vi "_list_CSM documented VIs.vi"(11 "Only CSM Folder":bool=TRUE) -> (3 "Array":path[](array[path]))   [LabVIEW 2017, in "csmdoc.lvlib"]
uses:
  csmdoc.lvlib
  _Shared/CSM Shared.lvlib
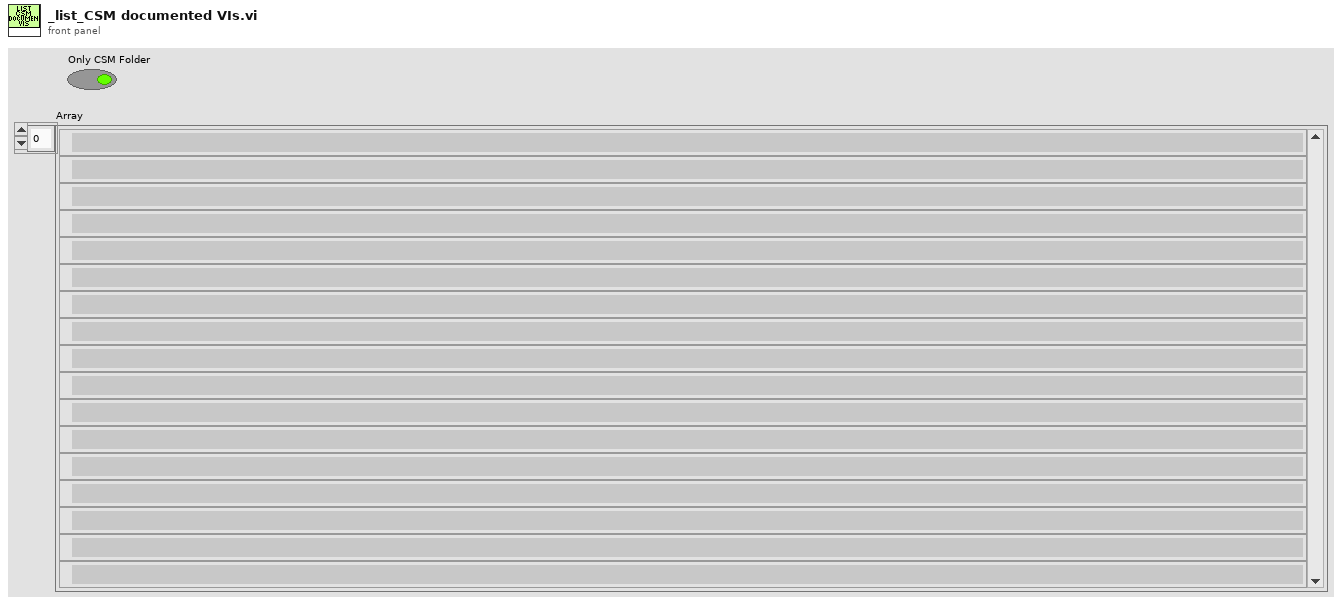
[diagram p1: front panel]
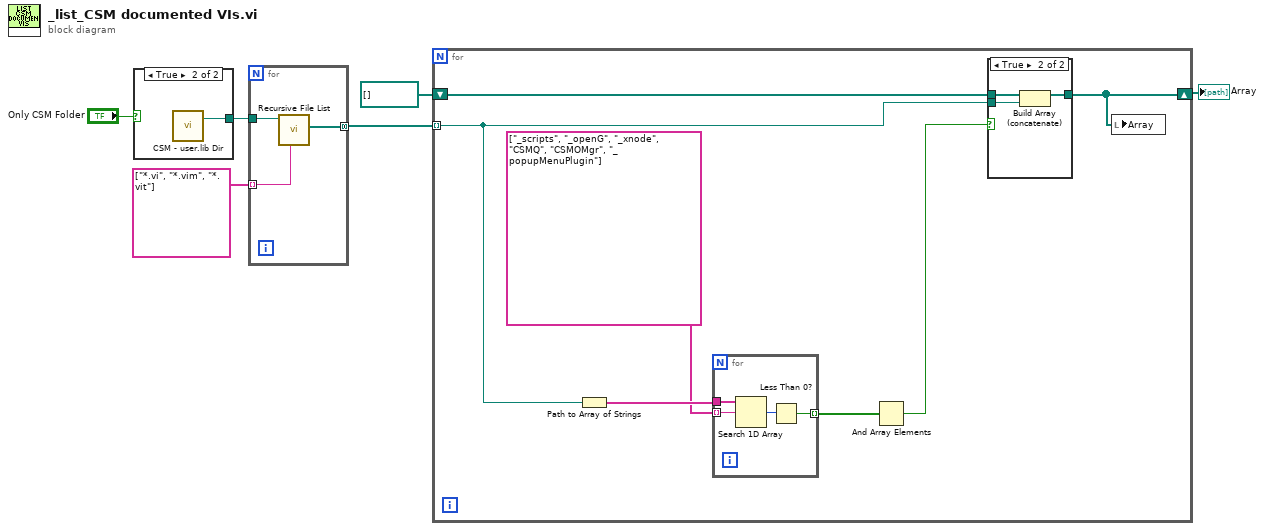
[diagram p0: block diagram]
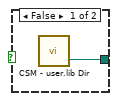
[diagram p2: hidden frame]
diagram:
  n1 = case shown="True" "Only CSM Folder" {
    tunnel: [w7 w8] -> w4
    frame False {
      n2 = call "CSM - user.lib Dir.vi"() -> ("<LabVIEW>"=w7:path)  [unwired: 2 in, 1 out]
    }
    frame True {
      n3 = call "CSM - user.lib Dir.vi"() -> ("csm_user.lib_dir"=w8:path)  [unwired: 2 in, 1 out]
    }
  }
  n4 = for {
    tunnel: w4 -> [w11]
    tunnel: string[] ["*.vi", "*.vim", "*.vit"] -> [w10] mode=indexing
    tunnel: [w9] -> w5 mode=concatenating
    n5 = call <vilib>:"Recursive File List.vi"("pattern"=w10, "Folder Path"=w11) -> ("All Files in Dir"=w9:path[])  [unwired: 5 in, 4 out]
  }
  n6 = for {
    tunnel: w5 -> [w17] mode=indexing
    shift-right: [w16] -> w2
    shift-left: path[] [] ("All Files in Dir") -> [w18]
    n7 = Path to Array of Strings(0:w17) -> (2:w15:string[])  [unwired: 1 out]
    n8 = for {
      tunnel: w15 -> [w22]
      tunnel: string[] ["_scripts", "_openG", "_xnode", "CSMQ", "CSMOMgr", "_popupMenuPlugin"] ("element") -> [w21] mode=indexing
      tunnel: [w19] -> w13 mode=indexing
      n9 = Search 1D Array(1D array=w22, element=w21) -> (index of element=w20:i32)  [unwired: 1 in]
      n10 = Less Than 0?(x=w20) -> (x < 0?=w19:bool)
    }
    n11 = And Array Elements(Boolean array=w13) -> (logical AND=w12:bool)
    n12 = case shown="True" w12 {
      tunnel: w18 -> [w23 w26]
      tunnel: [w23 w25] -> w16
      tunnel: w17 -> [_ w24]
      frame False {
      }
      frame True {
        n13 = Build Array (concatenate)(w26, w24) -> (w25:path[])
      }
    }
    n14 = local write "Array"(w16) -> ()
  }
  "Array" <- w2
